vi "Read Channel Names.vi"(8 "error in (no error)":errorcluster, 11 "Lakeshore 218 in":refnum<class "Lakeshore 218.lvclass">) -> (0 "error out":errorcluster, 2 "Channel Names":string[](array[string])=["Telescope RA", "Telescope DEC", "Telescope Moving?", "Telescope Status"], 3 "Lakeshore 218 out":refnum<class "Lakeshore 218.lvclass">)   [LabVIEW 2022 SP3, in "Lakeshore 218.lvclass"]
uses:
  Lakeshore 218.lvclass
  Lakeshore 218.lvclass/Lakeshore 218.ctl
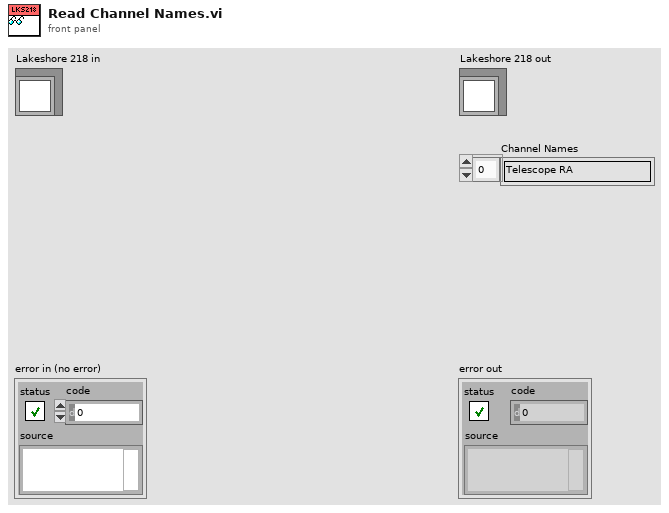
[diagram p1: front panel]
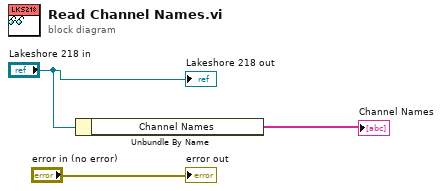
[diagram p0: block diagram]
diagram:
  n1 = Unbundle By Name("Lakeshore 218 in") -> ("Channel Names"=→"Channel Names":string[])
  "error out" <- "error in (no error)"
  "Lakeshore 218 out" <- "Lakeshore 218 in"
